vi "Test_ps3000e.vi"(7 "Channels":T7={"Channel A Settings "={"Enabled"=TRUE, "Coupling"=1, "Range"=8, "Analogue Offset"=0.0, "BandWidth"=0, "PROBE_RANGE_INFO"=1}, "Channel B Settings "={"Enabled"=TRUE, "Coupling"=1, "Range"=8, "Analogue Offset"=0.0, "BandWidth"=0, "PROBE_RANGE_INFO"=10}, "Channel C Settings "={"Enabled"=FALSE, "Coupling"=1, "Range"=8, "Analogue Offset"=0.0, "BandWidth"=0, "PROBE_RANGE_INFO"=1}, "Channel D Settings "={"Enabled"=FALSE, "Coupling"=1, "Range"=8, "Analogue Offset"=0.0, "BandWidth"=0, "PROBE_RANGE_INFO"=1}, "Channel E Settings "={"Enabled"=FALSE, "Coupling"=50, "Range"=5, "Analogue Offset"=0.0, "BandWidth"=0, "PROBE_RANGE_INFO"=0}, "Channel F Settings "={"Enabled"=FALSE, "Coupling"=50, "Range"=5, "Analogue Offset"=0.0, "BandWidth"=0, "PROBE_RANGE_INFO"=0}, "Channel G Settings "={"Enabled"=FALSE, "Coupling"=50, "Range"=5, "Analogue Offset"=0.0, "BandWidth"=0, "PROBE_RANGE_INFO"=0}, "Channel H Settings "={"Enabled"=FALSE, "Coupling"=50, "Range"=5, "Analogue Offset"=0.0, "BandWidth"=0, "PROBE_RANGE_INFO"=0}} {"Channel H Settings"."PROBE_RANGE_INFO" items=["PROBE_NONE_NV"=0, "X1_PROBE_NV"=1, "X10_PROBE_NV"=10]; "Channel H Settings"."BandWidth" items=["Full"=0, "100kHz"=100000, "20kHz"=200000, "1MHz"=1000000, "20MHz"=20000000, "25MHz"=25000000, "50MHz"=50000000, "200MHz"=200000000, "250MHz"=250000000, "500MHz"=500000000]; "Channel H Settings"."Range" items=["10mV"=0, "20mV"=1, "50mV"=2, "100mV"=3, "200mV"=4, "500mV"=5, "1V"=6, "2V"=7, "5V"=8, "10V"=9, "20V"=10, "50V"=11, "100V"=12, "200V"=13, "x10_Probe_100mV"=32, "x10_Probe_200mV"=33, "x10_Probe_500mV"=34, "x10_Probe_1V"=35, "x10_Probe_2V"=36, "x10_Probe_5V"=37, "x10_Probe_10V"=38, "x10_Probe_20V"=39, "x10_Probe_50V"=40, "x10_Probe_100V"=41, "x10_Probe_200V"=42, "x10_Probe_500V"=43, "CURRENT_CLAMP_60A_2A"=10500, "CURRENT_CLAMP_60A_5A"=10501, "CURRENT_CLAMP_60A_10A"=10502, "CURRENT_CLAMP_60A_20A"=10503, "CURRENT_CLAMP_60A_50A"=10504, "CURRENT_CLAMP_60A_60A"=10505, "CURRENT_CLAMP_60A_V2_0_5A"=10600, "CURRENT_CLAMP_60A_V2_1A"=10601, "CURRENT_CLAMP_60A_V2_2A"=10602, "CURRENT_CLAMP_60A_V2_5A"=10603, "CURRENT_CLAMP_60A_V2_10A"=10604, "CURRENT_CLAMP_60A_V2_20A"=10605, "CURRENT_CLAMP_60A_V2_50A"=10606, "CURRENT_CLAMP_60A_V2_60A"=10607, "RESISTANCE_LEAD_NEG5_TO_20OHM"=7000, "RESISTANCE_LEAD_NEG50_TO_200OHM"=7001, "RESISTANCE_LEAD_NEG500_TO_2KOHM"=7002, "RESISTANCE_LEAD_NEG5K_TO_20KOHM"=7003, "RESISTANCE_LEAD_NEG50K_TO_LEAD_200KOHM"=7004, "RESISTANCE_LEAD_NEG500K_TO_LEAD_2MOHM"=7005, "RESISTANCE_LEAD_DIODE_TEST"=7006, "HT_NEG3_TO_5KV"=8950, "HT_NEG3_TO_10KV"=8951, "HT_NEG5_TO_20KV"=8952, "HT_NEG5_TO_50KV"=8953, "HT_NEG5_TO_100KV"=8954, "HT_NEG3_TO_5KV_INVERTED"=8955, "HT_NEG3_TO_10KV_INVERTED"=8956, "HT_NEG5_TO_20KV_INVERTED"=8957, "HT_NEG5_TO_50KV_INVERTED"=8958, "HT_NEG5_TO_100KV_INVERTED"=8959, "TEMPERATURE_NEG50_TO_150DEGC"=9000, "PRESSURE_SENSOR_-100k-150k_PASCALS"=9100, "PRESSURE_SENSOR_-100k_TO_400k_PASCALS"=9101, "PRESSURE_SENSOR_-200k_TO_800k_PASCALS"=9102, "PRESSURE_SENSOR_-400k_TO_1600k_PASCALS"=9103, "PRESSURE_SENSOR_-400k_TO_3400k_PASCALS"=9104, "PRESSURE_SENSOR_-150k_TO_1350k_PASCALS"=9105]; "Channel H Settings"."Coupling" items=["AC"=0, "DC 1M Ohm"=1, "DC 50 Ohm"=50]; "Channel G Settings"."PROBE_RANGE_INFO" items=["PROBE_NONE_NV"=0, "X1_PROBE_NV"=1, "X10_PROBE_NV"=10]; "Channel G Settings"."BandWidth" items=["Full"=0, "100kHz"=100000, "20kHz"=200000, "1MHz"=1000000, "20MHz"=20000000, "25MHz"=25000000, "50MHz"=50000000, "200MHz"=200000000, "250MHz"=250000000, "500MHz"=500000000]; "Channel G Settings"."Range" items=["10mV"=0, "20mV"=1, "50mV"=2, "100mV"=3, "200mV"=4, "500mV"=5, "1V"=6, "2V"=7, "5V"=8, "10V"=9, "20V"=10, "50V"=11, "100V"=12, "200V"=13, "x10_Probe_100mV"=32, "x10_Probe_200mV"=33, "x10_Probe_500mV"=34, "x10_Probe_1V"=35, "x10_Probe_2V"=36, "x10_Probe_5V"=37, "x10_Probe_10V"=38, "x10_Probe_20V"=39, "x10_Probe_50V"=40, "x10_Probe_100V"=41, "x10_Probe_200V"=42, "x10_Probe_500V"=43, "CURRENT_CLAMP_60A_2A"=10500, "CURRENT_CLAMP_60A_5A"=10501, "CURRENT_CLAMP_60A_10A"=10502, "CURRENT_CLAMP_60A_20A"=10503, "CURRENT_CLAMP_60A_50A"=10504, "CURRENT_CLAMP_60A_60A"=10505, "CURRENT_CLAMP_60A_V2_0_5A"=10600, "CURRENT_CLAMP_60A_V2_1A"=10601, "CURRENT_CLAMP_60A_V2_2A"=10602, "CURRENT_CLAMP_60A_V2_5A"=10603, "CURRENT_CLAMP_60A_V2_10A"=10604, "CURRENT_CLAMP_60A_V2_20A"=10605, "CURRENT_CLAMP_60A_V2_50A"=10606, "CURRENT_CLAMP_60A_V2_60A"=10607, "RESISTANCE_LEAD_NEG5_TO_20OHM"=7000, "RESISTANCE_LEAD_NEG50_TO_200OHM"=7001, "RESISTANCE_LEAD_NEG500_TO_2KOHM"=7002, "RESISTANCE_LEAD_NEG5K_TO_20KOHM"=7003, "RESISTANCE_LEAD_NEG50K_TO_LEAD_200KOHM"=7004, "RESISTANCE_LEAD_NEG500K_TO_LEAD_2MOHM"=7005, "RESISTANCE_LEAD_DIODE_TEST"=7006, "HT_NEG3_TO_5KV"=8950, "HT_NEG3_TO_10KV"=8951, "HT_NEG5_TO_20KV"=8952, "HT_NEG5_TO_50KV"=8953, "HT_NEG5_TO_100KV"=8954, "HT_NEG3_TO_5KV_INVERTED"=8955, "HT_NEG3_TO_10KV_INVERTED"=8956, "HT_NEG5_TO_20KV_INVERTED"=8957, "HT_NEG5_TO_50KV_INVERTED"=8958, "HT_NEG5_TO_100KV_INVERTED"=8959, "TEMPERATURE_NEG50_TO_150DEGC"=9000, "PRESSURE_SENSOR_-100k-150k_PASCALS"=9100, "PRESSURE_SENSOR_-100k_TO_400k_PASCALS"=9101, "PRESSURE_SENSOR_-200k_TO_800k_PASCALS"=9102, "PRESSURE_SENSOR_-400k_TO_1600k_PASCALS"=9103, "PRESSURE_SENSOR_-400k_TO_3400k_PASCALS"=9104, "PRESSURE_SENSOR_-150k_TO_1350k_PASCALS"=9105]; "Channel G Settings"."Coupling" items=["AC"=0, "DC 1M Ohm"=1, "DC 50 Ohm"=50]; "Channel F Settings"."PROBE_RANGE_INFO" items=["PROBE_NONE_NV"=0, "X1_PROBE_NV"=1, "X10_PROBE_NV"=10]; "Channel F Settings"."BandWidth" items=["Full"=0, "100kHz"=100000, "20kHz"=200000, "1MHz"=1000000, "20MHz"=20000000, "25MHz"=25000000, "50MHz"=50000000, "200MHz"=200000000, "250MHz"=250000000, "500MHz"=500000000]; "Channel F Settings"."Range" items=["10mV"=0, "20mV"=1, "50mV"=2, "100mV"=3, "200mV"=4, "500mV"=5, "1V"=6, "2V"=7, "5V"=8, "10V"=9, "20V"=10, "50V"=11, "100V"=12, "200V"=13, "x10_Probe_100mV"=32, "x10_Probe_200mV"=33, "x10_Probe_500mV"=34, "x10_Probe_1V"=35, "x10_Probe_2V"=36, "x10_Probe_5V"=37, "x10_Probe_10V"=38, "x10_Probe_20V"=39, "x10_Probe_50V"=40, "x10_Probe_100V"=41, "x10_Probe_200V"=42, "x10_Probe_500V"=43, "CURRENT_CLAMP_60A_2A"=10500, "CURRENT_CLAMP_60A_5A"=10501, "CURRENT_CLAMP_60A_10A"=10502, "CURRENT_CLAMP_60A_20A"=10503, "CURRENT_CLAMP_60A_50A"=10504, "CURRENT_CLAMP_60A_60A"=10505, "CURRENT_CLAMP_60A_V2_0_5A"=10600, "CURRENT_CLAMP_60A_V2_1A"=10601, "CURRENT_CLAMP_60A_V2_2A"=10602, "CURRENT_CLAMP_60A_V2_5A"=10603, "CURRENT_CLAMP_60A_V2_10A"=10604, "CURRENT_CLAMP_60A_V2_20A"=10605, "CURRENT_CLAMP_60A_V2_50A"=10606, "CURRENT_CLAMP_60A_V2_60A"=10607, "RESISTANCE_LEAD_NEG5_TO_20OHM"=7000, "RESISTANCE_LEAD_NEG50_TO_200OHM"=7001, "RESISTANCE_LEAD_NEG500_TO_2KOHM"=7002, "RESISTANCE_LEAD_NEG5K_TO_20KOHM"=7003, "RESISTANCE_LEAD_NEG50K_TO_LEAD_200KOHM"=7004, "RESISTANCE_LEAD_NEG500K_TO_LEAD_2MOHM"=7005, "RESISTANCE_LEAD_DIODE_TEST"=7006, "HT_NEG3_TO_5KV"=8950, "HT_NEG3_TO_10KV"=8951, "HT_NEG5_TO_20KV"=8952, "HT_NEG5_TO_50KV"=8953, "HT_NEG5_TO_100KV"=8954, "HT_NEG3_TO_5KV_INVERTED"=8955, "HT_NEG3_TO_10KV_INVERTED"=8956, "HT_NEG5_TO_20KV_INVERTED"=8957, "HT_NEG5_TO_50KV_INVERTED"=8958, "HT_NEG5_TO_100KV_INVERTED"=8959, "TEMPERATURE_NEG50_TO_150DEGC"=9000, "PRESSURE_SENSOR_-100k-150k_PASCALS"=9100, "PRESSURE_SENSOR_-100k_TO_400k_PASCALS"=9101, "PRESSURE_SENSOR_-200k_TO_800k_PASCALS"=9102, "PRESSURE_SENSOR_-400k_TO_1600k_PASCALS"=9103, "PRESSURE_SENSOR_-400k_TO_3400k_PASCALS"=9104, "PRESSURE_SENSOR_-150k_TO_1350k_PASCALS"=9105]; "Channel F Settings"."Coupling" items=["AC"=0, "DC 1M Ohm"=1, "DC 50 Ohm"=50]; "Channel E Settings"."PROBE_RANGE_INFO" items=["PROBE_NONE_NV"=0, "X1_PROBE_NV"=1, "X10_PROBE_NV"=10]; "Channel E Settings"."BandWidth" items=["Full"=0, "100kHz"=100000, "20kHz"=200000, "1MHz"=1000000, "20MHz"=20000000, "25MHz"=25000000, "50MHz"=50000000, "200MHz"=200000000, "250MHz"=250000000, "500MHz"=500000000]; "Channel E Settings"."Range" items=["10mV"=0, "20mV"=1, "50mV"=2, "100mV"=3, "200mV"=4, "500mV"=5, "1V"=6, "2V"=7, "5V"=8, "10V"=9, "20V"=10, "50V"=11, "100V"=12, "200V"=13, "x10_Probe_100mV"=32, "x10_Probe_200mV"=33, "x10_Probe_500mV"=34, "x10_Probe_1V"=35, "x10_Probe_2V"=36, "x10_Probe_5V"=37, "x10_Probe_10V"=38, "x10_Probe_20V"=39, "x10_Probe_50V"=40, "x10_Probe_100V"=41, "x10_Probe_200V"=42, "x10_Probe_500V"=43, "CURRENT_CLAMP_60A_2A"=10500, "CURRENT_CLAMP_60A_5A"=10501, "CURRENT_CLAMP_60A_10A"=10502, "CURRENT_CLAMP_60A_20A"=10503, "CURRENT_CLAMP_60A_50A"=10504, "CURRENT_CLAMP_60A_60A"=10505, "CURRENT_CLAMP_60A_V2_0_5A"=10600, "CURRENT_CLAMP_60A_V2_1A"=10601, "CURRENT_CLAMP_60A_V2_2A"=10602, "CURRENT_CLAMP_60A_V2_5A"=10603, "CURRENT_CLAMP_60A_V2_10A"=10604, "CURRENT_CLAMP_60A_V2_20A"=10605, "CURRENT_CLAMP_60A_V2_50A"=10606, "CURRENT_CLAMP_60A_V2_60A"=10607, "RESISTANCE_LEAD_NEG5_TO_20OHM"=7000, "RESISTANCE_LEAD_NEG50_TO_200OHM"=7001, "RESISTANCE_LEAD_NEG500_TO_2KOHM"=7002, "RESISTANCE_LEAD_NEG5K_TO_20KOHM"=7003, "RESISTANCE_LEAD_NEG50K_TO_LEAD_200KOHM"=7004, "RESISTANCE_LEAD_NEG500K_TO_LEAD_2MOHM"=7005, "RESISTANCE_LEAD_DIODE_TEST"=7006, "HT_NEG3_TO_5KV"=8950, "HT_NEG3_TO_10KV"=8951, "HT_NEG5_TO_20KV"=8952, "HT_NEG5_TO_50KV"=8953, "HT_NEG5_TO_100KV"=8954, "HT_NEG3_TO_5KV_INVERTED"=8955, "HT_NEG3_TO_10KV_INVERTED"=8956, "HT_NEG5_TO_20KV_INVERTED"=8957, "HT_NEG5_TO_50KV_INVERTED"=8958, "HT_NEG5_TO_100KV_INVERTED"=8959, "TEMPERATURE_NEG50_TO_150DEGC"=9000, "PRESSURE_SENSOR_-100k-150k_PASCALS"=9100, "PRESSURE_SENSOR_-100k_TO_400k_PASCALS"=9101, "PRESSURE_SENSOR_-200k_TO_800k_PASCALS"=9102, "PRESSURE_SENSOR_-400k_TO_1600k_PASCALS"=9103, "PRESSURE_SENSOR_-400k_TO_3400k_PASCALS"=9104, "PRESSURE_SENSOR_-150k_TO_1350k_PASCALS"=9105]; "Channel E Settings"."Coupling" items=["AC"=0, "DC 1M Ohm"=1, "DC 50 Ohm"=50]; "Channel D Settings"."BandWidth" items=["Full"=0, "100kHz"=100000, "20kHz"=200000, "1MHz"=1000000, "20MHz"=20000000, "25MHz"=25000000, "50MHz"=50000000, "100MHz"=100000000, "200MHz"=200000000, "250MHz"=250000000, "350MHz"=350000000, "500MHz"=500000000]; "Channel D Settings"."PROBE_RANGE_INFO" items=["PROBE_NONE_NV"=0, "X1_PROBE_NV"=1, "X10_PROBE_NV"=10]; "Channel D Settings"."Range" items=["10mV", "20mV", "50mV", "100mV", "200mV", "500mV", "1V", "2V", "5V", "10V", "20V", "50V", "100V", "200V"]; "Channel D Settings"."Coupling" items=["AC"=0, "DC 1M Ohm"=1, "DC 50 Ohm"=50]; "Channel C Settings"."BandWidth" items=["Full"=0, "100kHz"=100000, "20kHz"=200000, "1MHz"=1000000, "20MHz"=20000000, "25MHz"=25000000, "50MHz"=50000000, "100MHz"=100000000, "200MHz"=200000000, "250MHz"=250000000, "350MHz"=350000000, "500MHz"=500000000]; "Channel C Settings"."PROBE_RANGE_INFO" items=["PROBE_NONE_NV"=0, "X1_PROBE_NV"=1, "X10_PROBE_NV"=10]; "Channel C Settings"."Range" items=["10mV", "20mV", "50mV", "100mV", "200mV", "500mV", "1V", "2V", "5V", "10V", "20V", "50V", "100V", "200V"]; "Channel C Settings"."Coupling" items=["AC"=0, "DC 1M Ohm"=1, "DC 50 Ohm"=50]; "Channel B Settings"."BandWidth" items=["Full"=0, "100kHz"=100000, "20kHz"=200000, "1MHz"=1000000, "20MHz"=20000000, "25MHz"=25000000, "50MHz"=50000000, "100MHz"=100000000, "200MHz"=200000000, "250MHz"=250000000, "350MHz"=350000000, "500MHz"=500000000]; "Channel B Settings"."PROBE_RANGE_INFO" items=["PROBE_NONE_NV"=0, "X1_PROBE_NV"=1, "X10_PROBE_NV"=10]; "Channel B Settings"."Range" items=["10mV", "20mV", "50mV", "100mV", "200mV", "500mV", "1V", "2V", "5V", "10V", "20V", "50V", "100V", "200V"]; "Channel B Settings"."Coupling" items=["AC"=0, "DC 1M Ohm"=1, "DC 50 Ohm"=50]; "Channel A Settings"."PROBE_RANGE_INFO" items=["PROBE_NONE_NV"=0, "X1_PROBE_NV"=1, "X10_PROBE_NV"=10]; "Channel A Settings"."Range" items=["10mV", "20mV", "50mV", "100mV", "200mV", "500mV", "1V", "2V", "5V", "10V", "20V", "50V", "100V", "200V"]; "Channel A Settings"."BandWidth" items=["Full"=0, "100kHz"=100000, "20kHz"=200000, "1MHz"=1000000, "20MHz"=20000000, "25MHz"=25000000, "50MHz"=50000000, "100MHz"=100000000, "200MHz"=200000000, "250MHz"=250000000, "350MHz"=350000000, "500MHz"=500000000]; "Channel A Settings"."Coupling" items=["AC"=0, "DC 1M Ohm"=1, "DC 50 Ohm"=50]}, 8 "Trigger Settings":T4={"Trigger Enabled"=TRUE, "Trigger Threshold (Volts)"=0.5, "Trigger Direction"=2, "Trigger Delay (samples)"=0, "Auto Trigger Time (us)"=1000000, "Trigger Source"=0} {"Trigger Source" items=["Channel A"=0, "Channel B"=1, "Channel C"=2, "Channel D"=3, "Channel E"=4, "Channel F"=5, "Channel G"=6, "Channel H"=7, "Port 0"=128, "Port 1"=129, "Trigger AUX"=1001]; "Auto Trigger Time (us)" format="%.4p"; "Trigger Direction" items=["Above", "Below", "Rising", "Falling", "Rising or Falling"]; "Trigger Threshold (Volts)" format="%#_6p"}, 9 "Acquisition Settings":T2={"preTriggerSamples"=0, "postTriggerSamples"=150000, "timebase"=2} {"postTriggerSamples" format="%_6p"; "preTriggerSamples" format="%_6p"}, 10 "Buffer and Transfer Settings":T3={"startIndex"=0, "Samples"=10000, "Down Sample Ratio"=16, "Down-Sample Mode"=2} {"Down-Sample Mode" items=["RAW none"=2147483648, "None"=0, "Aggregate"=1, "Decimate"=2, "Average"=4]; "Down Sample Ratio" step=1; "Samples" format="%_6p"}) -> (11 "Analog Channels":cluster{i32, dbl, "Data":dbl[]}[](graph)=[{0, 3.19488e-05, "Data"=[0.9882583170254402, 1.0176125244618395, 0.9980430528375733, 1.0176125244618395, 0.9882583170254402, 0.9980430528375733, 0.9882583170254402, 0.9882583170254402, 1.0078277886497065, 0.9882583170254402, 1.0078277886497065, 0.9882583170254402, 1.0078277886497065, 1.0078277886497065, 1.0078277886497065, 0.9980430528375733, 0.9882583170254402, 0.9784735812133072, 1.0078277886497065, 1.0078277886497065, 0.9882583170254402, 1.0078277886497065, 1.0273972602739725, 0.9882583170254402, 0.9980430528375733, 0.9980430528375733, 1.0078277886497065, 1.0176125244618395, 0.9882583170254402, 0.9980430528375733, 0.9980430528375733, 0.9980430528375733, 1.0176125244618395, 0.9980430528375733, 0.9980430528375733, 0.9882583170254402, 0.9882583170254402, 0.9882583170254402, 1.0078277886497065, 1.0273972602739725, 1.0176125244618395, 1.0078277886497065, 0.9980430528375733, 0.9980430528375733, 0.9784735812133072, 0.9980430528375733, 0.9882583170254402, 1.0078277886497065, 0.9882583170254402, 1.0078277886497065, 0.9980430528375733, 0.9882583170254402, 0.9882583170254402, 0.9882583170254402, 0.9882583170254402, 0.9882583170254402, 0.9882583170254402, 0.9980430528375733, 1.0176125244618395, 0.9980430528375733, 0.9980430528375733, 0.9980430528375733, 1.0078277886497065, 1.0078277886497065, 1.0273972602739725, 0.9882583170254402, 1.0176125244618395, 0.9882583170254402, 1.0078277886497065, 0.9882583170254402, 0.9980430528375733, 0.9980430528375733, 0.9882583170254402, 0.9980430528375733, 0.9980430528375733, 1.0078277886497065, 0.9882583170254402, 1.0078277886497065, 1.0078277886497065, 0.009784735812133072, -0.029354207436399216, 0.009784735812133072, -0.009784735812133072, -0.009784735812133072, -0.04892367906066536, 0.0, -0.009784735812133072, 0.009784735812133072, -0.019569471624266144, 0.029354207436399216, -0.009784735812133072, 0.009784735812133072, -0.029354207436399216, 0.0, 0.0, 0.0, -0.009784735812133072, -0.029354207436399216, -0.009784735812133072, 0.0, 0.0, 0.009784735812133072, 0.009784735812133072, -0.009784735812133072, -0.009784735812133072, 0.0, 0.0, 0.009784735812133072, 0.0, -0.03913894324853229, 0.0, -0.009784735812133072, 0.0, 0.009784735812133072, -0.009784735812133072, 0.0, -0.009784735812133072, 0.019569471624266144, -0.009784735812133072, -0.029354207436399216, 0.0, 0.0, 0.009784735812133072, -0.019569471624266144, 0.0, -0.019569471624266144, -0.009784735812133072, 0.0, -0.009784735812133072, 0.009784735812133072, 0.009784735812133072, -0.009784735812133072, 0.0, -0.009784735812133072, 0.0, -0.019569471624266144, 0.019569471624266144, -0.029354207436399216, -0.019569471624266144, -0.019569471624266144, 0.019569471624266144, 0.019569471624266144, 0.009784735812133072, 0.009784735812133072, 0.0, 0.0, 0.0, 0.0, -0.019569471624266144, 0.029354207436399216, 0.009784735812133072, -0.019569471624266144, 0.009784735812133072, -0.019569471624266144, -0.019569471624266144, -0.009784735812133072, 0.009784735812133072, 1.0176125244618395, 0.9980430528375733, 1.0176125244618395, 0.9980430528375733, 0.9882583170254402, 0.9980430528375733, 1.0078277886497065, 0.9980430528375733, 0.9882583170254402, 1.0078277886497065, 0.9980430528375733, 0.9882583170254402, 1.0078277886497065, 0.9980430528375733, 1.0078277886497065, 1.0176125244618395, 0.9980430528375733, 0.9784735812133072, 0.9980430528375733, 0.9784735812133072, 1.0078277886497065, 0.9980430528375733, 0.9784735812133072, 1.0078277886497065, 0.9784735812133072, 0.9980430528375733, 0.9980430528375733, 0.9980430528375733, 0.9491193737769079, 0.9882583170254402, 0.9882583170254402, 0.9784735812133072, 0.9980430528375733, 0.9784735812133072, 0.9784735812133072, 0.9980430528375733, 0.958904109589041, 0.9980430528375733, 1.0176125244618395, 0.9882583170254402, 0.9980430528375733, 0.9784735812133072, 0.9980430528375733, 0.9980430528375733, 0.9980430528375733, 0.9882583170254402, 0.9980430528375733, 0.9686888454011742, 1.0078277886497065, 0.9784735812133072, 1.0078277886497065, 1.0078277886497065, 0.9980430528375733, 0.9980430528375733, 1.0078277886497065, 0.9882583170254402, 1.0078277886497065, 1.0078277886497065, 0.9882583170254402, 1.0176125244618395, 0.9980430528375733, 0.9882583170254402, 1.0078277886497065, 0.9980430528375733, 0.9882583170254402, 0.9882583170254402, 0.9980430528375733, 0.9980430528375733, 0.9980430528375733, 0.9980430528375733, 0.9980430528375733, 1.0176125244618395, 0.9784735812133072, 0.9980430528375733, 0.9784735812133072, 0.9980430528375733, 0.9784735812133072, 1.0176125244618395, -0.019569471624266144, 0.009784735812133072, 0.0, 0.009784735812133072, -0.019569471624266144, -0.019569471624266144, -0.009784735812133072, 0.009784735812133072, -0.009784735812133072, -0.029354207436399216, -0.03913894324853229, -0.019569471624266144, -0.03913894324853229, -0.029354207436399216, -0.019569471624266144, -0.019569471624266144, -0.019569471624266144, 0.0, -0.019569471624266144, 0.0, 0.019569471624266144, 0.0, -0.03913894324853229, -0.019569471624266144, 0.019569471624266144, 0.019569471624266144, -0.009784735812133072, 0.019569471624266144, 0.009784735812133072, -0.009784735812133072, -0.009784735812133072, -0.019569471624266144, -0.019569471624266144, 0.0, -0.029354207436399216, 0.0, 0.0, 0.009784735812133072, -0.009784735812133072, -0.019569471624266144, 0.0, 0.0, 0.009784735812133072, -0.009784735812133072, -0.03913894324853229, -0.009784735812133072, -0.03913894324853229, -0.009784735812133072, 0.0, -0.019569471624266144, 0.009784735812133072, 0.029354207436399216, -0.029354207436399216, -0.009784735812133072, 0.0, 0.019569471624266144, 0.0, -0.029354207436399216, -0.019569471624266144, 0.0, -0.029354207436399216, 0.0, -0.04892367906066536, -0.019569471624266144, 0.0, -0.019569471624266144, -0.03913894324853229, -0.009784735812133072, 0.019569471624266144, -0.009784735812133072, -0.04892367906066536, -0.029354207436399216, 0.019569471624266144, -0.03913894324853229, -0.009784735812133072, -0.03913894324853229, -0.029354207436399216, -0.009784735812133072, 0.9980430528375733, 1.0078277886497065, 1.0078277886497065, 0.9784735812133072, 0.9980430528375733, 0.9882583170254402, 0.9980430528375733, 0.9882583170254402, 0.9980430528375733, 1.0078277886497065, 1.0176125244618395, 0.9882583170254402, 0.9980430528375733, 0.9882583170254402, 1.0078277886497065, 0.9882583170254402, 1.0078277886497065, 0.9882583170254402, 1.0176125244618395, 0.9882583170254402, 1.0078277886497065, 0.9784735812133072, 0.9784735812133072, 1.0078277886497065, 0.9980430528375733, 1.0273972602739725, 1.0273972602739725, 0.9784735812133072, 0.9980430528375733, 1.0078277886497065, 0.9882583170254402, 0.9882583170254402, 0.9882583170254402, 0.9784735812133072, 0.9882583170254402, 1.0176125244618395, 0.9882583170254402, 0.9882583170254402, 0.9882583170254402, 0.9980430528375733, 1.0176125244618395, 1.0078277886497065, 1.0078277886497065, 1.0078277886497065, 0.9980430528375733, 0.9980430528375733, 0.9784735812133072, 0.9882583170254402, 0.9980430528375733, 0.9980430528375733, 0.9882583170254402, 0.9980430528375733, 0.9980430528375733, 1.0078277886497065, 0.9980430528375733, 1.0176125244618395, 0.9784735812133072, 0.9980430528375733, 1.0176125244618395, 1.0176125244618395, 0.9686888454011742, 0.9784735812133072, 0.9980430528375733, 1.0078277886497065, 1.0176125244618395, 0.9882583170254402, 1.0078277886497065, 0.9980430528375733, 0.9980430528375733, 1.0078277886497065, 0.9980430528375733, 1.0273972602739725, 0.9882583170254402, 1.0176125244618395, 0.9882583170254402, 1.0078277886497065, 0.9784735812133072, 1.0078277886497065, 0.9686888454011742, -0.009784735812133072, -0.009784735812133072, 0.0, 0.009784735812133072, -0.03913894324853229, 0.0, 0.0, 0.019569471624266144, 0.029354207436399216, 0.0, 0.029354207436399216, 0.019569471624266144, 0.009784735812133072, 0.009784735812133072, 0.019569471624266144, 0.009784735812133072, 0.0, 0.0, -0.019569471624266144, 0.0, -0.019569471624266144, -0.009784735812133072, -0.009784735812133072, 0.0, -0.009784735812133072, 0.009784735812133072, -0.019569471624266144, -0.009784735812133072, 0.0, 0.029354207436399216, 0.0, -0.019569471624266144, -0.03913894324853229, -0.019569471624266144, 0.009784735812133072, 0.019569471624266144, -0.009784735812133072, -0.009784735812133072, 0.0, 0.009784735812133072, -0.019569471624266144, -0.019569471624266144, 0.009784735812133072, 0.019569471624266144, 0.0, 0.0, 0.0, 0.009784735812133072, -0.03913894324853229, -0.019569471624266144, -0.019569471624266144, -0.009784735812133072, -0.009784735812133072, -0.019569471624266144, -0.009784735812133072, 0.0, -0.009784735812133072, -0.029354207436399216, -0.009784735812133072, -0.03913894324853229, -0.019569471624266144, 0.0, 0.0, -0.009784735812133072, -0.019569471624266144, 0.009784735812133072, -0.019569471624266144, 0.0, -0.019569471624266144, -0.009784735812133072, -0.019569471624266144, 0.0, -0.009784735812133072, 0.0, -0.019569471624266144, 0.0, 0.019569471624266144, -0.03913894324853229, 0.9784735812133072, 0.9980430528375733, 0.9980430528375733, 0.9980430528375733, 0.9882583170254402, 1.0176125244618395, 0.9980430528375733, 0.9980430528375733, 1.0176125244618395, 0.9784735812133072, 0.9882583170254402, 0.9980430528375733, 0.9980430528375733, 0.9882583170254402, 0.9980430528375733, 1.0273972602739725, 1.0078277886497065, 1.0273972602739725, 0.9980430528375733, 1.0078277886497065, 0.9980430528375733, 1.0078277886497065, 1.0078277886497065, 0.9882583170254402, 0.9882583170254402, 0.9882583170254402, 0.9980430528375733, 1.0176125244618395, 1.0078277886497065, 0.9980430528375733, 1.0176125244618395, 0.9882583170254402, 0.9882583170254402, 0.9980430528375733, 0.9980430528375733, 1.0078277886497065, 1.0078277886497065, 0.9882583170254402, 1.0176125244618395, 0.9980430528375733, 0.9980430528375733, 0.9882583170254402, 0.9980430528375733, 1.0176125244618395, 0.9980430528375733, 1.0078277886497065, 1.0078277886497065, 1.0078277886497065, 1.0078277886497065, 1.0078277886497065, 1.0078277886497065, 1.0078277886497065, 1.0078277886497065, 0.9980430528375733, 0.9882583170254402, 0.9980430528375733, 1.0078277886497065, 0.9980430528375733, 1.0078277886497065, 1.0078277886497065, 0.9980430528375733, 0.9784735812133072, 1.0078277886497065, 1.0078277886497065, 0.9980430528375733, 0.9980430528375733, 1.0078277886497065, 0.9882583170254402, 0.9882583170254402, 1.0078277886497065, 0.9882583170254402, 0.9980430528375733, 0.9784735812133072, 0.9882583170254402, 1.0078277886497065, 0.9980430528375733, 1.0078277886497065, 1.0078277886497065, 0.029354207436399216, 0.0, 0.019569471624266144, 0.0, 0.009784735812133072, 0.009784735812133072, -0.019569471624266144, 0.009784735812133072, 0.009784735812133072, 0.009784735812133072, 0.0, -0.019569471624266144, -0.009784735812133072, -0.019569471624266144, 0.0, 0.009784735812133072, -0.009784735812133072, 0.009784735812133072, 0.0, 0.03913894324853229, -0.019569471624266144, 0.0, 0.009784735812133072, 0.0, 0.0, -0.009784735812133072, -0.009784735812133072, -0.029354207436399216, 0.009784735812133072, 0.029354207436399216, -0.009784735812133072, 0.0, -0.019569471624266144, 0.0, 0.0, 0.009784735812133072, 0.009784735812133072, 0.0, -0.009784735812133072, 0.019569471624266144, 0.0, -0.009784735812133072, 0.0, 0.009784735812133072, 0.009784735812133072, 0.0, 0.0, -0.019569471624266144, 0.0, -0.019569471624266144, 0.0, 0.009784735812133072, -0.009784735812133072, -0.009784735812133072, 0.0, 0.0, 0.009784735812133072, -0.009784735812133072, -0.019569471624266144, -0.029354207436399216, 0.0, 0.0, 0.0, -0.03913894324853229, 0.019569471624266144, 0.009784735812133072, 0.019569471624266144, 0.009784735812133072, -0.03913894324853229, 0.0, 0.019569471624266144, 0.009784735812133072, -0.009784735812133072, 0.009784735812133072, -0.009784735812133072, -0.009784735812133072, 0.23238747553816047]}, ...(4 in all)])   [LabVIEW 2024]
uses:
  Treiber_und_SubVis/PicoScopepsospaLib/PicoScopeospaAnalogChannelSettings.ctl
  Treiber_und_SubVis/PicoScopepsospaLib/PicoScopeospaDigitalChannelSettings.ctl
  Treiber_und_SubVis/shared/Buffer and Transfer Settings.ctl
  Treiber_und_SubVis/shared/Acquisition Settings.ctl
  Treiber_und_SubVis/shared/PicoBuffers.ctl
  <vilib>/Waveform/DWDTOps.llb/DWDT Analog to Digital.vi
panel:
  out "error read_buff":errorcluster
  in  "Reset":bool
  in  "handle in":i16=16384
  out "Pico psospa Units":string
  out "Device Info":T1={"PICO_DRIVER_VERSION"="psospa Windows Driver, 1.0.158.5815", "PICO_USB_VERSION"="3.0", "PICO_HARDWARE_VERSION"="1.0", "PICO_VARIANT_INFO"="3417EMSO", "PICO_BATCH_AND_SERIAL"="12667/0028", "PICO_CAL_DATE"="28Oct25", "PICO_KERNEL_VERSION"="1", "PICO_DIGITAL_HARDWARE_VERSION"="0", "PICO_ANALOGUE_HARDWARE_VERSION"="1.11.0.0", "PICO_FIRMWARE_VERSION_1"="2.2.2.0", "PICO_FIRMWARE_VERSION_2"="0", "PICO_IPP_VERSION"="F:\\Picoscope3000e\\Scope_LabView\\ps3000e\\Treiber_und_SubVis\\psospa.dll", "PICO_DRIVER_PATH"="", "PICO_FIRMWARE_VERSION_3"="", "PICO_FRONT_PANEL_FIRMWARE_VERSION"="", "Number of Channels"=4, "MSO"=TRUE}
  in  "Resolution":u32(ring)=10 items=["8-bit"=0, "12-bit"=1, "14-bit"=2, "15-bit"=3, "16-bit"=4, "10-bit"=10]
  in  "error in (no error)":errorcluster
  in  "Digital Channels":T5={"Port 0 Settings "={"Enabled"=FALSE, "Threshold Level (Volts)"=1.0}, "Port 1 Settings"={"Enabled"=FALSE, "Threshold Level (Volts)"=1.0}} {"Port 1 Settings"."Threshold Level (Volts)" format="%#_4p"; "Port 0 Settings"."Threshold Level (Volts)" format="%#_4p"}
  out "Port 0":digitalwaveform(graph)={"t0"=timestamp(0 s since 1904-01-01), "dt"=3.19488e-05, "Y"={"transitions"=[], "data"=[]}}
  out "Properties Panel":T6={"Sample Frequency"=500801.282051282, "Sample Rate"=1.9968e-06, "Max Samples Available"=536870784, "Number of Samples"=0, "Total Capture Time (sec) "=0.0, "Max Total Capture Time Available (sec)"=1072.0235814912} {"Max Total Capture Time Available (sec)" format="%.3p"; "Sample Frequency" format="%.6p"; "Sample Rate" format="%.3p"; "Max Samples Available" format="%_6p"; "Total Capture Time (sec)" format="%.3p"}
  in  "timeIntervalRequested":dbl=2e-06 format="%#6_6p"
  # "D8-D15"
  # "DO-D7"
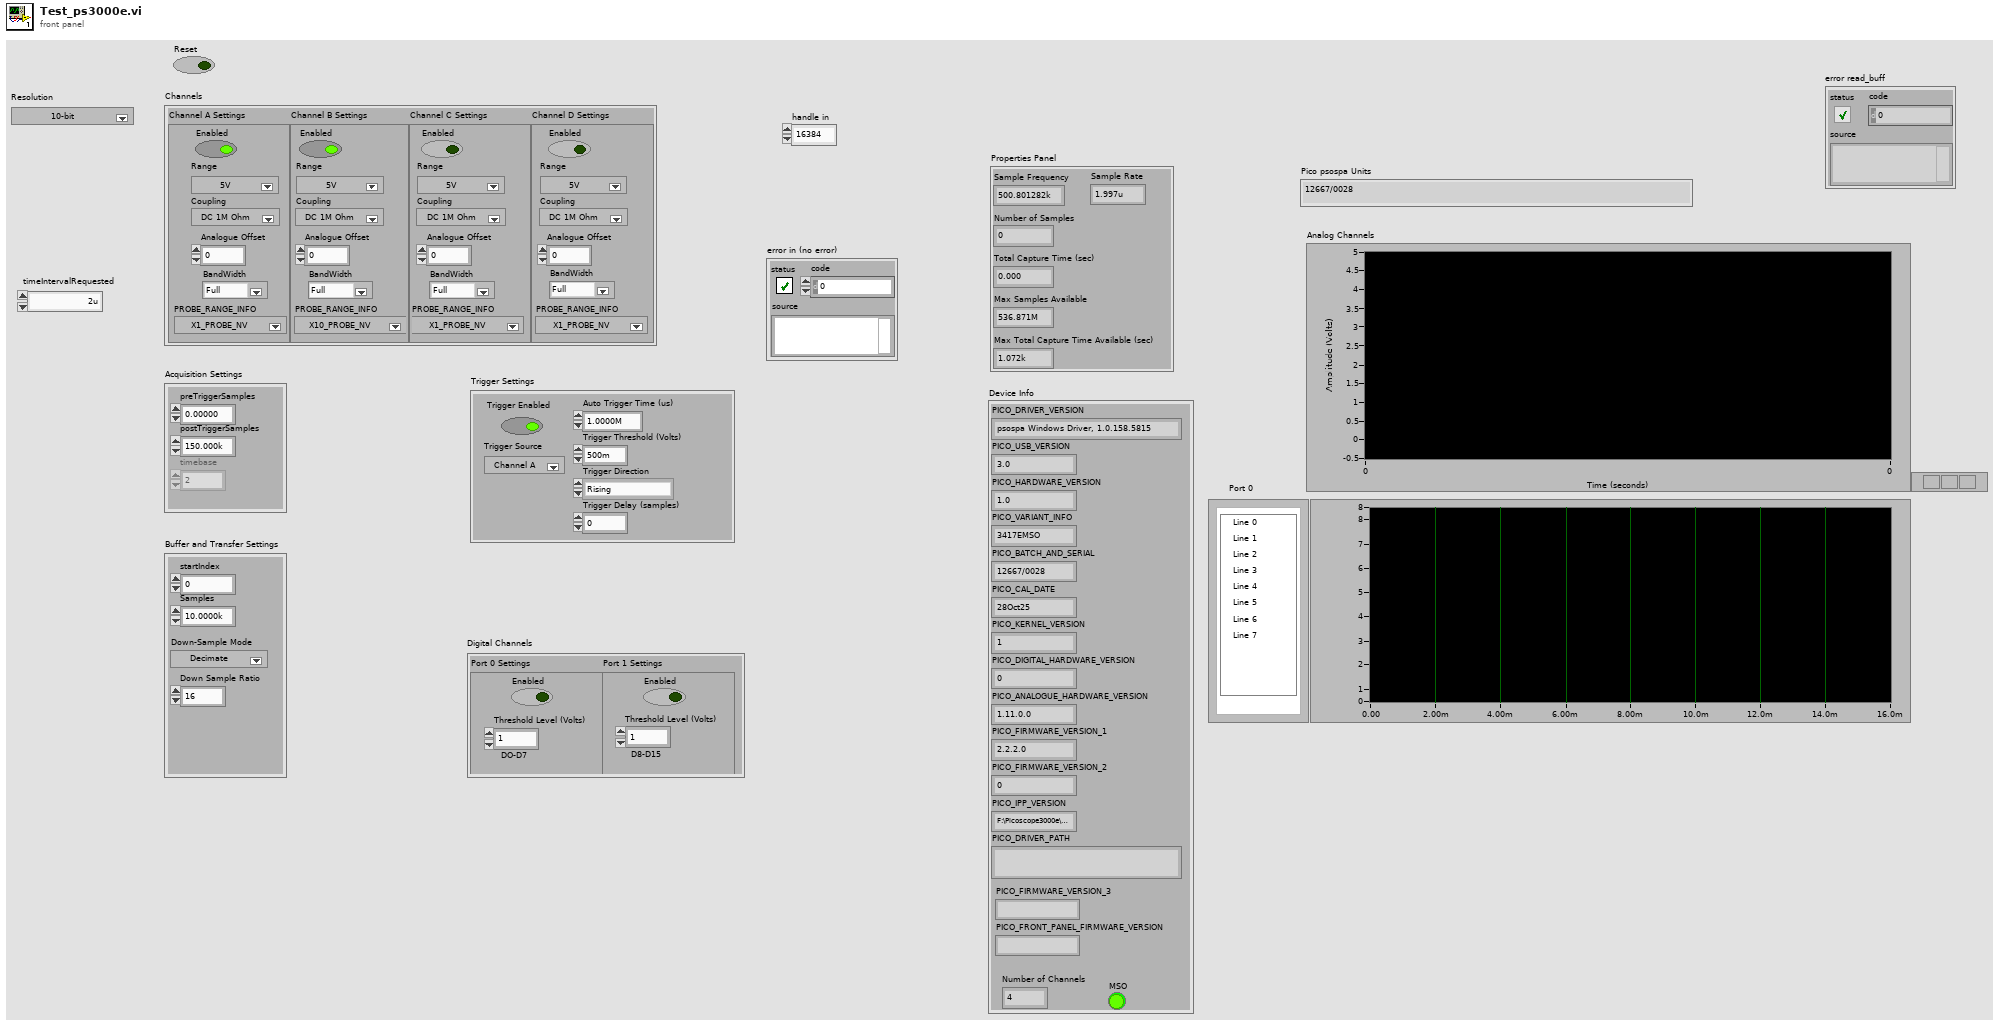
[diagram p1: front panel]
types:
  T1 = cluster{"PICO_DRIVER_VERSION":string, "PICO_USB_VERSION":string, "PICO_HARDWARE_VERSION":string, "PICO_VARIANT_INFO":string, "PICO_BATCH_AND_SERIAL":string, "PICO_CAL_DATE":string, "PICO_KERNEL_VERSION":string, "PICO_DIGITAL_HARDWARE_VERSION":string, "PICO_ANALOGUE_HARDWARE_VERSION":string, "PICO_FIRMWARE_VERSION_1":string, "PICO_FIRMWARE_VERSION_2":string, "PICO_IPP_VERSION":string, "PICO_DRIVER_PATH":string, "PICO_FIRMWARE_VERSION_3":string, "PICO_FRONT_PANEL_FIRMWARE_VERSION":string, "Number of Channels":i16, "MSO":bool}
  T2 = typedef "Acquisition Settings.ctl" = cluster{"preTriggerSamples":u64, "postTriggerSamples":u64, "timebase":u32}
  T3 = typedef "Buffer and Transfer Settings.ctl" = cluster{"startIndex":u64, "Samples":u64, "Down Sample Ratio":u64, "Down-Sample Mode":u32}
  T4 = cluster{"Trigger Enabled":bool, "Trigger Threshold (Volts)":dbl, "Trigger Direction":u16, "Trigger Delay (samples)":u64, "Auto Trigger Time (us)":u32, "Trigger Source":u32}
  T5 = typedef "PicoScopeospaDigitalChannelSettings.ctl" = cluster{"Port 0 Settings ":cluster{"Enabled":bool, "Threshold Level (Volts)":dbl}, "Port 1 Settings":cluster{"Enabled":bool, "Threshold Level (Volts)":dbl}}
  T6 = cluster{"Sample Frequency":dbl, "Sample Rate":dbl, "Max Samples Available":u64, "Number of Samples":u64, "Total Capture Time (sec) ":dbl, "Max Total Capture Time Available (sec)":dbl}
  T7 = typedef "PicoScopeospaAnalogChannelSettings.ctl" = cluster{"Channel A Settings ":cluster{"Enabled":bool, "Coupling":i16, "Range":u16, "Analogue Offset":dbl, "BandWidth":u32, "PROBE_RANGE_INFO":u32}, "Channel B Settings ":cluster{"Enabled":bool, "Coupling":i16, "Range":u16, "Analogue Offset":dbl, "BandWidth":u32, "PROBE_RANGE_INFO":u32}, "Channel C Settings ":cluster{"Enabled":bool, "Coupling":i16, "Range":u16, "Analogue Offset":dbl, "BandWidth":u32, "PROBE_RANGE_INFO":u32}, "Channel D Settings ":cluster{"Enabled":bool, "Coupling":i16, "Range":u16, "Analogue Offset":dbl, "BandWidth":u32, "PROBE_RANGE_INFO":u32}, "Channel E Settings ":cluster{"Enabled":bool, "Coupling":i16, "Range":u16, "Analogue Offset":dbl, "BandWidth":u32, "PROBE_RANGE_INFO":u32}, "Channel F Settings ":cluster{"Enabled":bool, "Coupling":i16, "Range":u16, "Analogue Offset":dbl, "BandWidth":u32, "PROBE_RANGE_INFO":u32}, "Channel G Settings ":cluster{"Enabled":bool, "Coupling":i16, "Range":u16, "Analogue Offset":dbl, "BandWidth":u32, "PROBE_RANGE_INFO":u32}, "Channel H Settings ":cluster{"Enabled":bool, "Coupling":i16, "Range":u16, "Analogue Offset":dbl, "BandWidth":u32, "PROBE_RANGE_INFO":u32}}
  T8 = typedef "PicoBuffers.ctl" = cluster{"Max Buffer Pointers":u64[][][], "Min Buffer Pointers":u64[][][], "StreamingDataInfo":cluster{"Channel":u32, "Down-Sample Mode":u32, "PICO_DATA_TYPE":enum32{"PICO_INT8_T", "PICO_INT16_T", "PICO_INT32_T", "PICO_UINT32_T", "PICO_INT64_T", ""}, "Samples":i32, "bufferIndex":u64, "startIndex":i32, "overflow":i16}[][]}
  T9 = cluster{"Channel A Buffer":i16[], "Channel B Buffer":i16[], "Channel C Buffer":i16[], "Channel D Buffer":i16[], "Channel E Buffer":i16[], "Channel F Buffer":i16[], "Channel G Buffer":i16[], "Channel H Buffer":i16[], "Port 0 Buffer":i16[], "Port 1 Buffer":i16[]}[]
  T10 = cluster{"Channel A Buffer":i16[], "Channel B Buffer":i16[], "Channel C Buffer":i16[], "Channel D Buffer":i16[], "Channel E Buffer":i16[], "Channel F Buffer":i16[], "Channel G Buffer":i16[], "Channel H Buffer":i16[], "Port 0 Buffer":i16[], "Port 1 Buffer":i16[]}
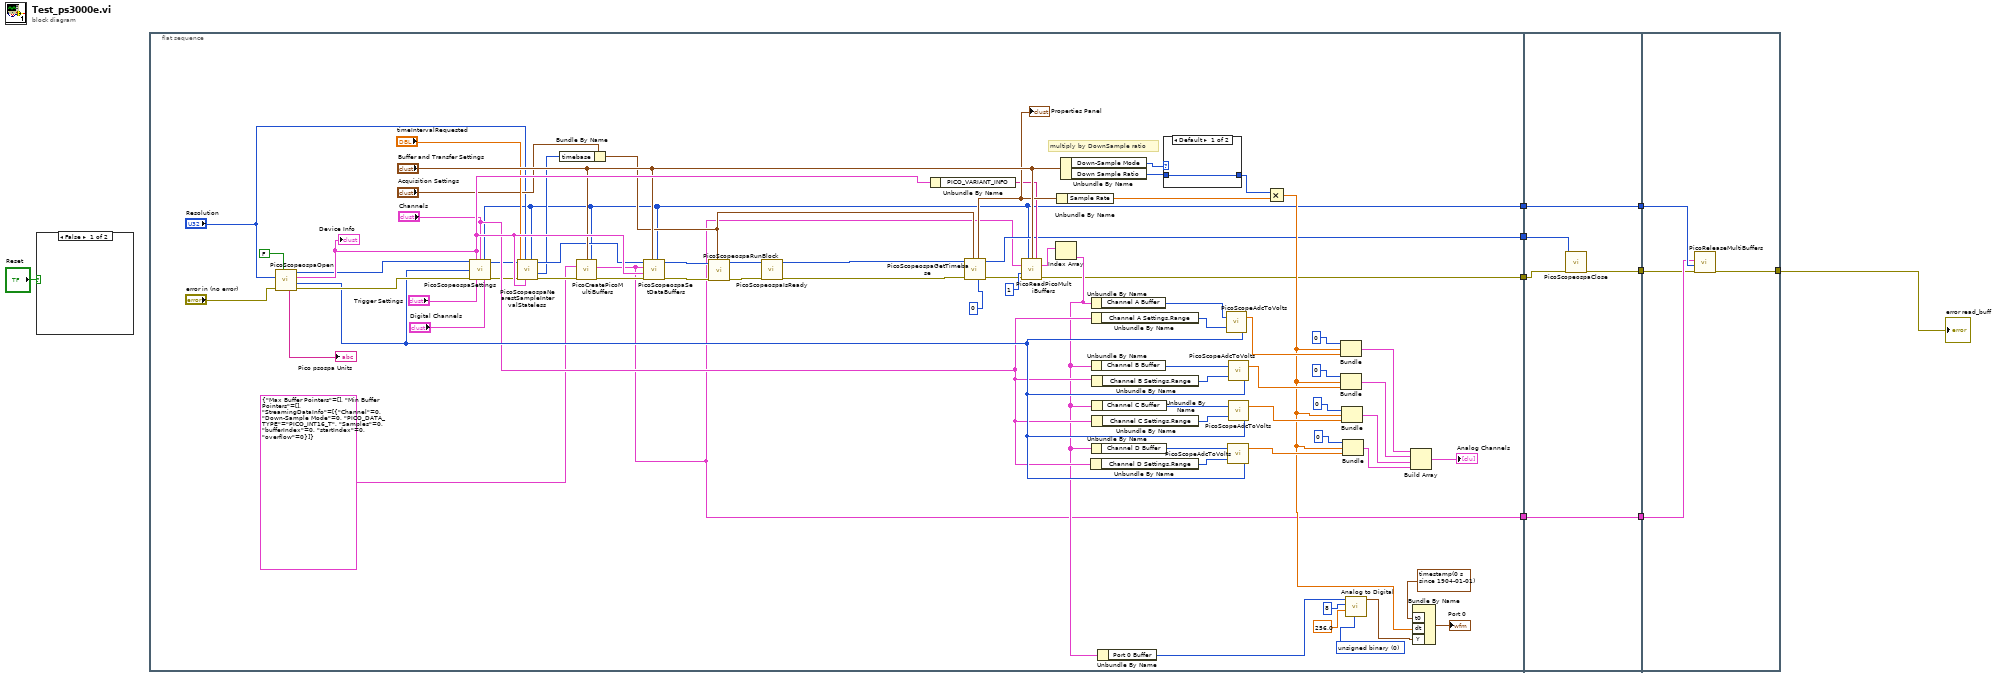
[diagram p0: block diagram]
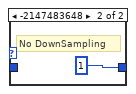
[diagram p2: hidden frame]
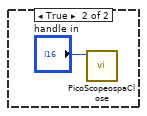
[diagram p3: hidden frame]
diagram:
  n1 = case shown="False" "Reset" {
    frame False {
    }
    frame True {
      n2 = call "PicoScopeospaClose.vi"("handle in"="handle in") -> ()  [unwired: 9 in, 2 out]
    }
  }
  n3 = flat-sequence {
    tunnel: [w18] -> w8
    tunnel: [w17] -> w7
    tunnel: [w16] -> w6
    tunnel: [w15] -> w5
    tunnel: w8 -> [w87]
    tunnel: w7 -> [w88]
    tunnel: w6 -> [w86]
    tunnel: w5 -> [w89]
    tunnel: [w89] -> w4
    tunnel: [w86] -> w2
    tunnel: [w85] -> w1
    tunnel: w4 -> [w91]
    tunnel: [w93] -> w3
    tunnel: w2 -> [w92]
    tunnel: w1 -> [w90]
    frame #0 {
      w42 = u16 0 items=["unsigned binary", "offset binary", "2's complement"] ("data format (offset binary)")
      # "multiply by DownSample ratio"
      n4 = call "PicoScopeospaOpen.vi"("Use Serial Number"=FALSE, "error in (no error)"="error in (no error)", "Resolution"="Resolution") -> ("error out"=w79:errorcluster, "Max ADC value"=w78:i16, "Device Info"=w80:T1, "handle out"=w11:i16, "psospa Units"=→"Pico psospa Units":string)  [unwired: 3 in, 1 out]
      "Device Info" <- w80
      n5 = call "PicoScopeospaSettings.vi"("handle in"=w11, "Device Info"=w80, "Channels"="Channels", "Max ADC value"=w78, "error in (no error)"=w79, "Trigger Settings"="Trigger Settings", "Digital Channels"="Digital Channels") -> ("Enabled array"=w16:i16[], "handle out"=w66:i16, "error out"=w69:errorcluster)  [unwired: 6 in]
      n6 = call "PicoScopeospaNearestSampleIntervalStateless.vi"("Enabled array"=w16, "Device Info"=w80, "Resolution"="Resolution", "error in (no error)"=w69, "timeIntervalRequested"="timeIntervalRequested", "handle in"=w66) -> ("error out"=w68:errorcluster, "timebase"=w62:u32, "handle out"=w67:i16)  [unwired: 2 in, 1 out]
      n7 = Bundle By Name(cluster="Acquisition Settings", "timebase"=w62) -> (w63:T2)
      n8 = call "PicoCreatePicoMultiBuffers.vi"("Buffer and Transfer Settings"="Buffer and Transfer Settings", "enabled array"=w16, "Data Pointers In"=T8 {"Max Buffer Pointers"=[], "Min Buffer Pointers"=[], "StreamingDataInfo"=[[{"Channel"=0, "Down-Sample Mode"=0, "PICO_DATA_TYPE"=enum."PICO_INT16_T", "Samples"=0, "bufferIndex"=0, "startIndex"=0, "overflow"=0}]]} ("Data Pointers"), "error in (no error)"=w68) -> ("Data Pointers"=w15:T8, "error out"=w74:errorcluster)  [unwired: 10 in]
      n9 = call "PicoScopeospaSetDataBuffers.vi"("enabled array"=w16, "Buffer and Transfer Settings"="Buffer and Transfer Settings", "error in (no error)"=w74, "Device Info"=w80, "Data Pointers In"=w15, "handle in"=w67) -> ("error out"=w73:errorcluster, "handle out"=w71:i16)  [unwired: 4 in]
      n10 = call "PicoScopeospaRunBlock.vi"("Acquisition Settings"=w63, "error in (no error)"=w73, "handle in"=w71) -> ("error out"=w28:errorcluster, "handle out"=w27:i16)  [unwired: 5 in, 2 out]
      n11 = call "PicoScopeospaIsReady.vi"("error in (no error)"=w28, "handle in"=w27) -> ("error out"=w13:errorcluster, "handle out"=w14:i16)  [unwired: 7 in, 1 out]
      n12 = Unbundle By Name(w80) -> ("PICO_VARIANT_INFO"=w24:string)
      n13 = call "PicoScopeospaGetTimebase.vi"("Number of Samples"=u64 0, "Acquisition Settings"=w63, "error in (no error)"=w13, "handle in"=w14) -> ("error out"=w23:errorcluster, "handle out"=w18:i16, "Properties Panel"=w30:T6)  [unwired: 5 in]
      "Properties Panel" <- w30
      n14 = call "PicoReadPicoMultiBuffers.vi"("enabled array"=w16, "Buffer and Transfer Settings"="Buffer and Transfer Settings", "Variant"=w24, "Data Pointers"=w15, "No of Buffers"=1, "error in (no error)"=w23) -> ("MultiBuffers (Max or non-aggregated)"=w35:T9, "error out"=w17:errorcluster)  [unwired: 7 in, 1 out]
      n15 = Index Array(array=w35) -> (element=w26:T10)  [unwired: 1 in]
      n16 = Unbundle By Name(w30) -> ("Sample Rate"=w33:dbl)
      n17 = Unbundle By Name("Buffer and Transfer Settings") -> ("Down-Sample Mode"=w31:u32, "Down Sample Ratio"=w32:u64)
      n18 = Unbundle By Name("Channels") -> ("Channel D Settings.Range"=w50:u16)
      n19 = Unbundle By Name(w26) -> ("Channel A Buffer"=w25:i16[])
      n20 = Unbundle By Name("Channels") -> ("Channel A Settings.Range"=w60:u16)
      n21 = Unbundle By Name(w26) -> ("Channel B Buffer"=w58:i16[])
      n22 = Unbundle By Name(w26) -> ("Channel D Buffer"=w51:i16[])
      n23 = Unbundle By Name("Channels") -> ("Channel B Settings.Range"=w57:u16)
      n24 = Unbundle By Name(w26) -> ("Channel C Buffer"=w53:i16[])
      n25 = Unbundle By Name("Channels") -> ("Channel C Settings.Range"=w52:u16)
      n26 = Unbundle By Name(w26) -> ("Port 0 Buffer"=w40:i16[])
      n27 = case shown="Default" w31 {
        tunnel: [w83 u64 1 ("Down Sample Ratio")] -> w29
        tunnel: w32 -> [w83 _]
        frame Default {
        }
        frame -2147483648 {
          # "No DownSampling"
        }
      }
      n28 = call "PicoScopeAdcToVolts.vi"("Max_adc"=w78, "Range Index"=w60, "Data"=w25) -> ("Data"=w36:dbl[])
      n29 = call "PicoScopeAdcToVolts.vi"("Max_adc"=w78, "Range Index"=w50, "Data"=w51) -> ("Data"=w46:dbl[])
      n30 = call "PicoScopeAdcToVolts.vi"("Max_adc"=w78, "Range Index"=w57, "Data"=w58) -> ("Data"=w56:dbl[])
      n31 = call "PicoScopeAdcToVolts.vi"("Max_adc"=w78, "Range Index"=w52, "Data"=w53) -> ("Data"=w47:dbl[])
      n32 = Multiply(x=w29, y=w33) -> (x*y=w22:dbl)
      n33 = Bundle(0, w22, "Data"=w36) -> (w55:cluster{i32, dbl, "Data":dbl[]})  [unwired: 1 in]
      n34 = Bundle(0, w22, "Data"=w56) -> (w54:cluster{i32, dbl, "Data":dbl[]})  [unwired: 1 in]
      n35 = Bundle(0, w22, "Data"=w47) -> (w45:cluster{i32, dbl, "Data":dbl[]})  [unwired: 1 in]
      n36 = Bundle(0, w22, "Data"=w46) -> (w44:cluster{i32, dbl, "Data":dbl[]})  [unwired: 1 in]
      n37 = call-poly <vilib>:"Analog to Digital.vi"("data format (offset binary)"=w42, "full-scale range (pk-pk)"=256.0, "resolution (16 bit)"=8, "analog waveform"=w40) -> ("digital waveform"=w37:digitalwaveform)  [unwired: 4 in, 3 out]
      n38 = Build Array(w55, w54, w45, w44) -> (→"Analog Channels":cluster{i32, dbl, "Data":dbl[]}[])
      n39 = Bundle By Name("t0"=timestamp(0 s since 1904-01-01), "dt"=w22, "Y"=w37) -> (→"Port 0":digitalwaveform)  [unwired: 1 in]
    }
    frame #1 {
      n40 = call "PicoScopeospaClose.vi"("error in (no error)"=w88, "handle in"=w87) -> ("error out"=w85:errorcluster)  [unwired: 8 in, 1 out]
    }
    frame #2 {
      n41 = call "PicoReleaseMultiBuffers.vi"("error in (no error)"=w90, "Enabled array"=w92, "Data Pointers"=w91) -> ("error out"=w93:errorcluster)  [unwired: 7 in, 1 out]
    }
  }
  "error read_buff" <- w3
